vi "SENS_IF_FREQ_M_A.vi"(0 "VISA IN":refnum<visa-resource-name>, 5 "error in":errorcluster, 7 "Channel":i32) -> (14 "VISA Out":refnum<visa-resource-name>, 16 "Data":string, 19 "error out":errorcluster)   [LabVIEW 2018, in "PNA-X.lvlib"]
doc: "SENSe<cnum>:IF:FREQuency? Min \n'returns the minimum allowable frequency setting \nReturn Type Numeric \nDefault 9 MHz \n1760\n\nLast Modified: \n18-Jan-2007 MX New topic \n1761\n\nSense:Mixer Commands \nPerforms Mixer setup and configuration. \nClick on a blue keyword to view the command details. \nSee Also \nExample Programs \nLearn about the Frequency Converter Application \nSynchronizing the PNA and Controller \nSCPI Command Tree \nSENSe<ch>:MIXer:APPLy \n(Write only) Applies the mixer setup settings and turns the channel ON. (Performs the same function \nas the Apply button on the mixer setup dialog box). \nParameters \n<ch> Any existing channel number. If unspecified, value is set to 1 \nExamples SENS:MIX:APPL \nQuery Syntax Not Applicable \nDefault Not Applicable \n1762\n\nSENSe<ch>:MIXer:AVOidspurs <bool> \n(Read Write) Sets and returns the state of the avoid spurs feature. Learn more about avoid spurs. \nParameters \n<ch> Any existing channel number. If unspecified, value is set to 1 \n<bool> Avoid spurs state. Choose from \n0 - Avoid spurs OFF \n1 - Avoid spurs ON \nExamples SENS:MIX:AVO \nsense2:mixer:avoidspurs 1 \nQuery Syntax SENSe<ch>:MIXer:AVOidspurs? \nReturn Type Boolean \nDefault 0 (OFF) \nSENSe<ch>:MIXer:CALCulate <char> \n(Write only) Calculates the Input, IF, or Output frequencies of the mixer setup and updates the \nchannel settings. \nParameters \n<ch> Any existing channel number. If unspecified, value is set to 1 \n<char> Mixer port to be calculated. Choose from: \n1763\n\n<char> 1st or only stage \nrequires: \nIn addition, 2nd stage \nrequires: \nINPUT \nOutput Start and Stop \nfrequencies \nLO frequency \nOutput sideband (High or \nLow) \nIF Start and Stop \nfrequencies \n2nd LO frequency \nIF sideband (High or Low) \nBoth NA \nIF Start and Stop \nfrequencies \nBoth LO frequencies \nOUTPUT \nInput Start and Stop \nfrequencies \nLO frequency \nOutput sideband (High or \nLow) \nIF Start and Stop \nfrequencies \n2nd LO frequency \nIF sideband (High or Low) \nLO_1 \nInput Start and Stop \nfrequencies \nOutput frequency \nOutput sideband (High or \nLow) \nIF Start and Stop \nfrequencies \n2nd LO frequency \nIF sideband (High or Low) \nLO_2 NA Input Start and stop \nfrequencies \n1st LO start and stop \nfrequencies \nOutput frequency \nIF sideband(High or Low \nOutput sideband(High or \nLow) \nExamples SENS:MIX:CALC Output \nQuery Syntax Not Applicable \nDefault Not Applicable \nSENSe<ch>:MIXer:LOAD <name> \n1764\n\n(Write-only) Loads a previously-configured mixer attributes file (.mxr) \nParameters \n<ch> Any existing channel number. If unspecified, value is set to 1. \n<name> Path and file name (including .mxr extension) to load. \nExamples SENSe:MIXer:LOAD \"C:\\Program Files\\Agilent\\Network \nAnalyzer\\Documents\\Mixer\\MyMixer.mxr\" \nDefault Not Applicable \nSENSe<ch>:MIXer:SAVE <name> \n(Write-only) Saves the settings for the mixer/converter test setup to a mixer attributes file. \nParameters \n<ch> Any existing channel number. If unspecified, value is set to 1. \n<name> Path and file name (including .mxr extension) to save. \nExamples SENSe:MIXer:SAVE \"C:\\Program Files\\Agilent\\Network \nAnalyzer\\Documents\\Mixer\\MyMixer.mxr\" \nDefault Not Applicable \nSENSe<ch>:MIXer:STAGe <n> \n(Read-Write) Number of IF stages of the mixer. \nParameters \n<ch> Any existing channel number. If unspecified, value is set to 1. \n<n> Number of stages. Choose either 1 or 2 \nExamples SENSe:MIX:STAG 2 \nSENSe:MIXer:STAGE 1 \nQuery Syntax SENSe<ch>:MIXer:STAGe? \nReturn Type Numeric \nDefault 1 \nSENSe<ch>:MIXer:IF:FREQuency:DENominator <num> \n1765\n\n(Read-Write) Sets or returns the denominator value of the IF Fractional Multiplier. \nParameters \n<ch> Any existing channel number. If unspecified, value is set to 1. \n<num> Denominator value. \nExamples SENSe:MIX:IF:FREQ:DEN 5 \nSENSe2:MIXer:IF:FREQ:DENominator 4 \nQuery Syntax SENSe<ch>:MIXer:IF:FREQuency:DENominator? \nReturn Type Numeric \nDefault Not Applicable \nSENSe<ch>:MIXer:IF:FREQuency:FIXed <num> \n(Read-Write) Sets or returns the fixed frequency of the IF.. \nParameters \n<ch> Any existing channel number. If unspecified, value is set to 1. \n<num> Frequency. \nExamples SENSe:MIXer:IF:FREQ:FIXed 1e9 \nSENSe2:MIXer:IF:FREQ:FIXed 1000000000 \nQuery Syntax SENSe<ch>:MIXer:IF:FREQuency:FIXed? \nReturn Type Numeric \nDefault Not Applicable \nSENSe<ch>:MIXer:IF:FREQuency:NUMerator <num> \n(Read-Write) Sets or returns the numerator value of the IF Fractional Multiplier. \nParameters \n<ch> Any existing channel number. If unspecified, value is set to 1. \n<num> Numerator value of the IF fractional multiplier \nExamples SENSe:MIX:IF:FREQ:NUM 4 \nSENSe2:MIXer:IF2:FREQ:NUMerator 3 \nQuery Syntax SENSe<ch>:MIXer:IF:FREQuency:NUMerator? \nReturn Type Numeric \nDefault Not Applicable \n1766\n\nSENSe<ch>:MIXer:IF:FREQuency:SIDeband <char> \n(Read-Write) Sets or returns the value of the IF sideband. \nParameters \n<ch> Any existing channel number. If unspecified, value is set to 1. \n<char> Sideband value. Choose from \nLOW - Low or Difference (-) \nHIGH - High or Sum (+) \nExamples SENS:MIX:IF:FREQ:SIDE LOW \nSENSe2:MIXer:IF:FREQ:SIDEband HIGH \nQuery Syntax SENSe<ch>:MIXer:IF:FREQuency:SIDeband? \nReturn Type Character \nDefault LOW \nSENSe<ch>:MIXer:IF:FREQuency:STARt <num> \n(Read-Write) Sets or returns the IF start frequency value of the mixer. \nParameters \n<ch> Any existing channel number. If unspecified, value is set to 1. \n<num> IF Start Frequency value \nExamples SENS:MIX:IF:FREQ:STAR 1e9 \nSENSe2:MIXer:IF:FREQ:STARt 1000000000 \nQuery Syntax SENSe<ch>:MIXer:IF:FREQuency:STARt? \nReturn Type Numeric \nDefault Not Applicable \nSENSe<ch>:MIXer:IF:FREQuency:STOP <num>\n1767\n\n(Read-Write) Sets or returns the stop frequency value of the mixer IF frequency. \nParameters \n<ch> Any existing channel number. If unspecified, value is set to 1. \n<num> IF Stop Frequency value \nExamples SENS:MIX:IF:FREQ:STOP 2e9 \nSENSe2:MIXer:IF:FREQ:STOP 2000000000 \nQuery Syntax SENSe<ch>:MIXer:IF:FREQuency:STOP? \nReturn Type Numeric \nDefault Not Applicable \nSENSe<ch>:MIXer:INPut:FREQuency:DENominator <value> \n(Read-Write) Sets or returns the denominator value of the Input Fractional Multiplier. \nParameters \n<ch> Any existing channel number. If unspecified, value is set to 1. \n<value> Input denominator value. \nExamples SENS:MIX:INP:FREQ:DEN 5 \nSENS2:MIXer:INPut:FREQ:DENominator 4 \nQuery Syntax SENSe<ch>:MIXer:INPut:FREQuency:DENominator? \nReturn Type Numeric \nDefault Not Applicable \nSENSe<ch>:MIXer:INPut:FREQuency:FIXed<value> \n(Read-Write) Sets or returns the fixed frequency of the input. \nParameters \n<ch> Any existing channel number. If unspecified, value is set to 1. \n<value> Input frequency. \nExamples SENSe:MIXer:INPut:FREQ:FIXed 1e9 \nSENSe2:MIXer:INPut:FREQ:FIXed 1000000000 \nQuery Syntax SENSe<ch>:MIXer:INPut:FREQuency:FIXed? \nReturn Type Numeric \nDefault Not Applicable \n1768\n\nSENSe<ch>:MIXer:INPut:FREQuency:MODE <char> \n(Read-Write) Sets or returns the Input sweep mode. \nParameters \n<ch> Any existing channel number. If unspecified, value is set to 1. \n<char> Input sweep mode. Choose either FIXED or SWEPT \nExamples SENS:MIX:INP:FREQ:MODE FIXED \nSENSe2:MIXer:INP:FREQ:MODE swept \nQuery Syntax SENSe<ch>:MIXer:INPut:FREQuency:MODE? \nReturn Type Character \nDefault Fixed \nSENSe<ch>:MIXer:INPut:FREQuency:NUMerator <value> \n(Read-Write) Sets or returns the numerator value of the Input Fractional Multiplier. \nParameters \n<ch> Any existing channel number. If unspecified, value is set to 1. \n<value> Input numerator value. \nExamples SENS:MIX:INP:FREQ:NUM 3 \nSENSe2:MIXer:INPut:FREQ:NUMerator 1 \nQuery Syntax SENSe<ch>:MIXer:INPut:FREQ:NUMerator? \nReturn Type Numeric \nDefault Not Applicable \nSENSe<ch>:MIXer:INPut:FREQuency:STARt <value> \n1769\n\n(Read-Write) Sets or returns the Input start frequency value of the mixer. \nParameters \n<ch> Any existing channel number. If unspecified, value is set to 1. \n<value> Input Start frequency \nExamples SENS:MIX:INP:FREQ:STAR 1e9 \nSENSe2:MIXer:INPut:FREQ:STARt 1000000000 \nQuery Syntax SENSe<ch>:MIXer:INPut:FREQuency:STARt? \nReturn Type Numeric \nDefault Not Applicable \nSENSe<ch>:MIXer:INPut:FREQuency:STOP <value> \n(Read-Write) Sets or returns the Input stop frequency value of the mixer. \nParameters \n<ch> Any existing channel number. If unspecified, value is set to 1. \n<value> Input stop frequency \nExamples SENS:MIX:INP:FREQ:STOP 2e9 \nSENSe2:MIXer:INPut:FREQ:STOP 2000000000 \nQuery Syntax SENSe<ch>:MIXer:INPut:FREQuency:STOP? \nReturn Type Numeric \nDefault Not Applicable \nSENSe<ch>:MIXer:INPut:POWer <value> \n(Read-Write) Sets or returns the value of the Input Power. \nParameters \n<ch> Any existing channel number. If unspecified, value is set to 1. \n<value> Input power in dBm. \nExamples SENS:MIX:INP:POW 9 \nSENSe2:MIXer:INPut:POWer 5 \nQuery Syntax SENSe<ch>:MIXer:INPut:POWer? \nReturn Type Numeric \nDefault Not Applicable \n1770\n\nSENSe<ch>:MIXer:INPut:POWer:USENominal <bool> \n(Read-Write) Toggles the Nominal Incident Power setting ON and OFF. This setting is ONLY to be \nused with SMC measurements, not VMC. Learn more about Nominal Incident Power. \nParameters \n<ch> Any existing channel number. If unspecified, value is set to 1. \n<value> (boolean) - Nominal Incident Power State. Choose from: \nTrue (1) - Turn nominal incident power ON \nFalse (0) - Turn nominal incident power OFF \nExamples SENS:MIX:INP:POW:USEN 1 \nSENSe2:MIXer:INPut:POWer:USENominal false \nQuery Syntax SENSe<ch>:MIXer:INPut:POWer:USENominal? \nReturn Type Boolean \nDefault False \nSENSe<ch>:MIXer:LO<n>:FREQuency:DENominator <value> \n(Read-Write) Sets or returns the denominator value of the LO Fractional Multiplier. \nParameters \n<ch> Any existing channel number. If unspecified, value is set to 1. \n<n> LO stage number. Choose 1 or 2. \n<value> LO denominator. \nExamples SENS:MIX:LO:FREQ:DEN 5 \nSENSe2:MIXer:LO2:FREQ:DENominator 4 \nQuery Syntax SENSe<ch>:MIXer:LO<n>:FREQuency:DENominator? \nReturn Type Numeric \nDefault 1 \nSENSe<ch>:MIXer:LO<n>:FREQuency:FIXed <value> \n1771\n\n(Read-Write) Sets or returns the fixed frequency of the specified mixer LO. \nParameters \n<ch> Any existing channel number. If unspecified, value is set to 1. \n<n> LO stage number. Choose 1 or 2 \n<value> LO frequency. \nExamples SENS:MIX:LO:FREQ:FIX 1e9 \nSENSe2:MIXer:LO2:FREQ:FIXed 1000000000 \nQuery Syntax SENSe<ch>:MIXer:LO<n>:FREQuency:FIXed? \nReturn Type Numeric \nDefault Not Applicable \nSENSe<ch>:MIXer:LO<n>:FREQuency:ILTI <bool> \n(Read-Write) Specifies whether to use the Input frequency that is greater than the LO or less than \nthe LO. To learn more, see the mixer setup dialog box help. \nParameters \n<ch> Any existing channel number. If unspecified, value is set to 1. \n<n> LO stage number. Choose 1 or 2 \n<bool> True (1) - Use the Input that is Greater than the specified LO. \nFalse (0) - Use the Input that is Less than the specified LO. \nExamples SENS:MIX:LO1:FREQ:ILTI 1 \nsense2:mixer:lo2:frequency:ilti true \nQuery Syntax SENSe<ch>:MIXer:LO<n>:FREQuency:ILTI? \nReturn Type Boolean \nDefault False \nSENSe<ch>:MIXer:LO<n>:FREQuency:MODE <char> \n1772\n\n(Read-Write) Sets or returns the LO sweep mode. \nParameters \n<ch> Any existing channel number. If unspecified, value is set to 1. \n<n> LO stage number. Choose 1 or 2 \n<char> LO sweep mode. Choose either FIXED or SWEPT \nExamples SENS:MIX:LO:FREQ:MODE FIXED \nSENSe2:MIXer:LO2:FREQ:MODE swept \nQuery Syntax SENSe<ch>:MIXer:LO<n>:FREQuency:MODE? \nReturn Type Character \nDefault Fixed \nSENSe<ch>:MIXer:LO<n>:FREQuency:NUMerator <value> \n(Read-Write) Sets or returns the numerator value of the LO Fractional Multiplier. \nParameters \n<ch> Any existing channel number. If unspecified, value is set to 1. \n<n> LO stage number. Choose 1 or 2 \n<value> LO Numerator. \nExamples SENS:MIX:LO:FREQ:NUM 5 \nSENSe2:MIXer:LO2:FREQ:NUMerator 4 \nQuery Syntax SENSe<ch>:MIXer:LO<n>:FREQuency:NUMerator? \nReturn Type Numeric \nDefault Not Applicable \nSENSe<ch>:MIXer:LO<n>:FREQuency:STARt <value> \n1773\n\n(Read-Write) Sets or returns the LO start frequency value. \nParameters \n<ch> Any existing channel number. If unspecified, value is set to 1. \n<n> LO stage number. Choose 1 or 2 \n<value> LO Start Frequency in Hertz. \nExamples SENS:MIX:LO:FREQ:STAR 5E9 \nQuery Syntax SENSe<ch>:MIXer:LO<n>:FREQuency:STARt? \nReturn Type Numeric \nDefault Not Applicable \nSENSe<ch>:MIXer:LO<n>:FREQuency:STOP <value> \n(Read-Write) Sets or returns the LO stop frequency value. \nParameters \n<ch> Any existing channel number. If unspecified, value is set to 1. \n<n> LO stage number. Choose 1 or 2 \n<value> LO Stop Frequency in Hertz. \nExamples SENS:MIX:LO:FREQ:STOP 5E9 \nQuery Syntax SENSe<ch>:MIXer:LO<n>:FREQuency:STOP? \nReturn Type Numeric \nDefault Not Applicable \nSENSe<ch>:MIXer:LO<n>:NAME <value> \n1774\n\n(Read-Write) Sets or returns the name of the previously-configured external LO source. The external \nLO source must be configured and calibrated manually; there are no programming commands to \naccomplish this. The source must also be properly connected. \nParameters \n<ch> Any existing channel number. If unspecified, value is set to 1. \n<n> LO stage number. Choose 1 or 2. \n<value> External LO source name \nExamples SENS:MIX:LO:NAME \"MySource\" \nQuery Syntax SENSe<ch>:MIXer:LO<n>:NAME? \nReturn Type String \nDefault Not Controlled \nSENSe<ch>:MIXer:LO<n>:POWer <value> \n(Read-Write) Sets or returns the value of the LO Power. \nParameters \n<ch> Any existing channel number. If unspecified, value is set to 1. \n<n> LO stage. Choose 1 or 2 \n<value> LO Power in dBm \nExamples SENS:MIX:LO:POW 9 \nQuery Syntax SENSe<ch>:MIXer:LO<n>:POWer? \nReturn Type Numeric \nDefault Not Applicable \nSENSe<ch>:MIXer:OUTPut:FREQuency:FIXed <value> \n1775\n\n(Read-Write) Sets or returns the output fixed frequency of the mixer. \nParameters \n<ch> Any existing channel number. If unspecified, value is set to 1. \n<value> Output fixed frequency in Hertz. \nExamples SENS:MIX:OUTP:FREQ:FIX 5e9 \nQuery Syntax SENSe<ch>:MIXer:OUTPut:FREQuency:FIXed? \nReturn Type Numeric \nDefault Not Applicable \nSENSe<ch>:MIXer:OUTPut:FREQuency:MODE <char> \n(Read-Write) Sets or returns the Output sweep mode. \nParameters \n<ch> Any existing channel number. If unspecified, value is set to 1. \n<char> Output sweep mode. Choose either FIXED or SWEPT \nExamples SENS:MIX:OUT:FREQ:MODE FIXED \nSENSe2:MIXer:OUTput:FREQuency:MODE swept \nQuery Syntax SENSe<ch>:MIXer:OUTPut:FREQuency:MODE? \nReturn Type Character \nDefault Fixed \nSENSe<ch>:MIXer:OUTPut:FREQuency:SIDeband <value> \n1776\n\n(Read-Write) Sets or returns the value of the output sideband. \nParameters \n<ch> Any existing channel number. If unspecified, value is set to 1. \n<value> Boolean Sideband value. Choose from \nLOW - Low or Difference (-) \nHIGH - High or Sum (+) \nExamples SENS:MIX:OUTP:FREQ:SIDe LOW \nSENSe2:MIXer:OUTPut:FREQ:SIDeband HIGH \nQuery Syntax SENSe<ch>:MIXer:OUTPut:FREQuency:SIDeband? \nReturn Type Character \nDefault LOW \nSENSe<ch>:MIXer:OUTPut:FREQuency:STARt <value> \n(Read-Write) Sets or returns the Output start frequency of the mixer. \nParameters \n<ch> Any existing channel number. If unspecified, value is set to 1. \n<value> Output start frequency \nExamples SENS:MIX:OUTP:FREQ:STAR 1e9 \nSENSe2:MIXer:OUTPut:FREQ:STARt 1000000000 \nQuery Syntax SENSe<ch>:MIXer:OUTPut:FREQuency:STARt? \nReturn Type Numeric \nDefault Not Applicable \nSENSe<ch>:MIXer:OUTPut:FREQuency:STOP <value> \n1777\n\n(Read-Write) Sets or returns the Output stop frequency of the mixer. \nParameters \n<ch> Any existing channel number. If unspecified, value is set to 1. \n<value> Output stop frequency \nExamples SENS:MIX:OUTP:FREQ:STOP 1e9 \nSENSe2:MIXer:OUTPut:FREQ:STOP 1000000000 \nQuery Syntax SENSe<ch>:MIXer:OUTPut:FREQuency:STOP? \nReturn Type Numeric \nDefault Not Applicable \n1778\n\nSense:Multiplexer Commands \nControls External Test Sets (N44xx, E5091A, and Special Opts). \nClick on a blue keyword to view the command details. \nRed commands are superseded. \nSee Also \nSee an example program using these commands. \nLearn about External Test Set Control \nSynchronizing the PNA and Controller \nSCPI Command Tree \nSENSe:MULTiplexer<id>:ADDRess <address> \n(Read-Write) Sets and returns the address for the external test set at the specified ID. This command \nshould be immediately preceded by the SENSe:MULT:TYPE command. \nParameters \n<id> Id of the external test set. If unspecified, Id is assumed to be 1. Must be \npreviously set by the SENSe:MULT:TYPE command. \n<address> Integer The test set address. \nFor a GPIB test set (N44xx and some specials), this is the GPIB address. \nFor a test set I/O test set (some specials), it is the position of the test set in the chain \n(starting at 0). \nFor USB test sets (E5091A), the address is set by DIP switches on the rear panel. \n1779\n\nExamples SENS:MULT1:TYPE \"Z5623A_K66\" ' use K66 test set, and reference it \nthrough ID 1 \nSENS:MULT1:ADDR 0 ' first test set in sequence \n' All subsequent commands using SENS:MULT1 will refer to this \ntest set \nQuery Syntax SENSe:MULTiplexer<id>:ADDRess? \nReturn Type Numeric \nDefault Not Applicable"
uses:
  PNA-X.lvlib
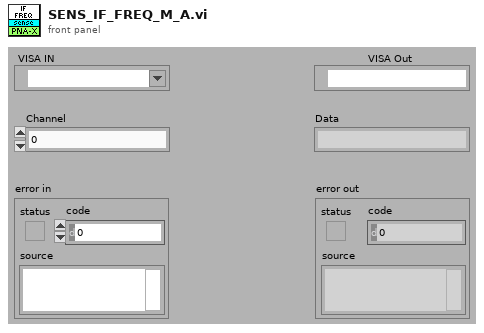
[diagram p1: front panel]
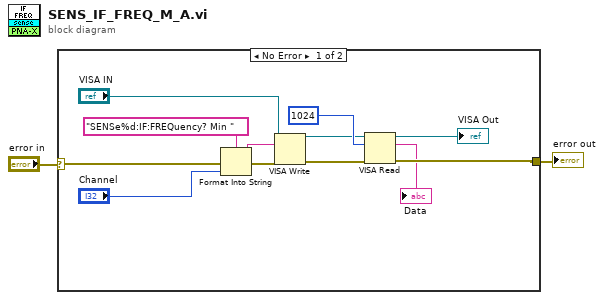
[diagram p0: block diagram]
diagram:
  n1 = case shown="No Error" "error in" {
    selector: "error in" -> [w14 w15]
    tunnel: [w5 w15] -> w1
    frame No Error {
      n2 = Format Into String(format string="SENSe%d:IF:FREQuency? Min " ("Cmdline"), error in=w14, "Channel") -> (resulting string=w12:string, error out=w13:errorcluster)  [unwired: 1 in]
      n3 = VISA Write(VISA resource name="VISA IN", write buffer=w12, error in (no error)=w13) -> (VISA resource name out=w7:refnum<visa-resource-name>, error out=w9:errorcluster)  [unwired: 1 out]
      n4 = VISA Read(VISA resource name=w7, byte count=1024, error in (no error)=w9) -> (VISA resource name out=→"VISA Out":refnum<visa-resource-name>, read buffer=→"Data":string, error out=w5:errorcluster)  [unwired: 1 out]
    }
    frame Error {
    }
  }
  "error out" <- w1
